vi "Timer.vi"(8 "error in (no error)":errorcluster, 11 "Message Queues in":T1) -> (0 "error out":errorcluster, 3 "Message Queue":refnum<queue>)   [LabVIEW 2014]
uses:
  support/Message Queue/All Message Queues.ctl
  support/Message Queue/Message Cluster.ctl
  Engine/Message.ctl
  support/Message Queue/Enqueue Message (Single).vi
  <vilib>/Utility/error.llb/Error Cluster From Error Code.vi
  <vilib>/ErrorRing/Error Ring.xnode
  support/Message Queue/Message Queue.lvlib
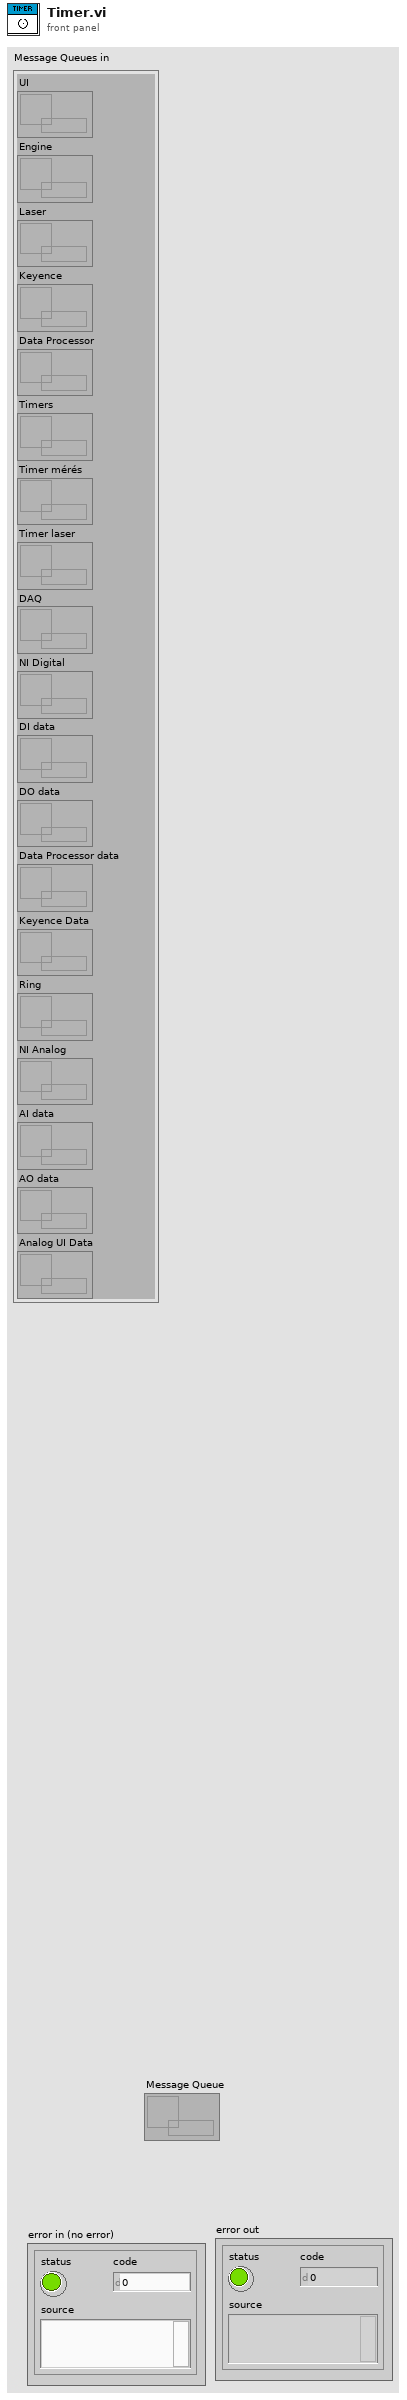
[diagram p1: front panel]
types:
  T1 = typedef "Message Queue.lvlib/All Message Queues.ctl" = cluster{"UI":refnum<queue>, "Engine":refnum<queue>, "Laser":refnum<queue>, "Keyence":refnum<queue>, "Data Processor":refnum<queue>, "Timers":refnum<queue>, "Timer mérés":refnum<queue>, "Timer laser":refnum<queue>, "DAQ":refnum<queue>, "NI Digital":refnum<queue>, "DI data":refnum<queue>, "DO data":refnum<queue>, "Data Processor data":refnum<queue>, "Keyence Data":refnum<queue>, "Ring":refnum<queue>, "NI Analog":refnum<queue>, "AI data":refnum<queue>, "AO data":refnum<queue>, "Analog UI Data":refnum<queue>}
  T2 = typedef "Message.ctl" = cluster{"Thread ID":u16, "Callback":string, "Data":variant, "Error":errorcluster}
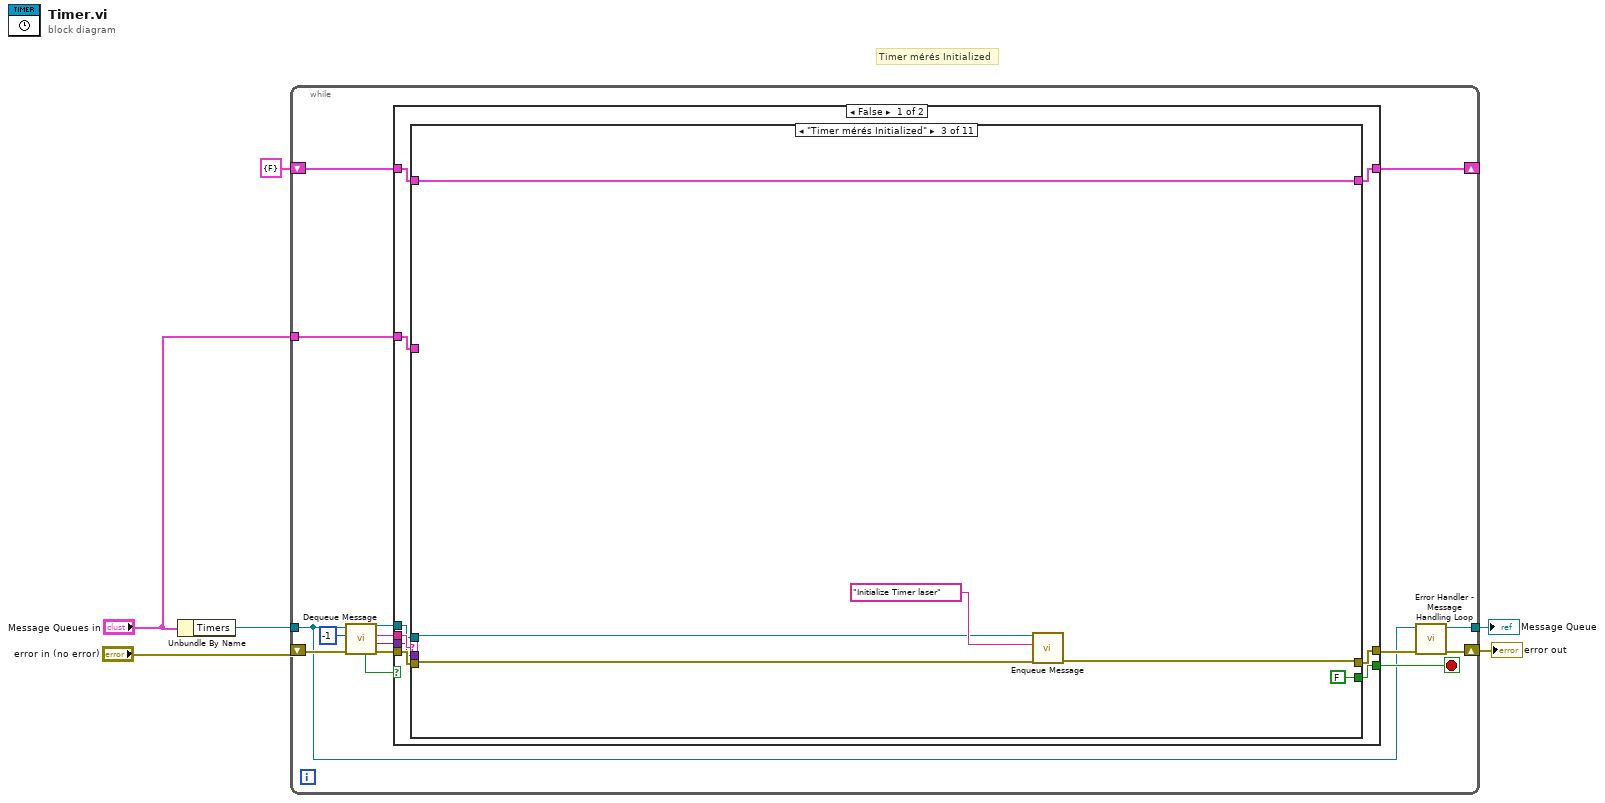
[diagram p0: block diagram]
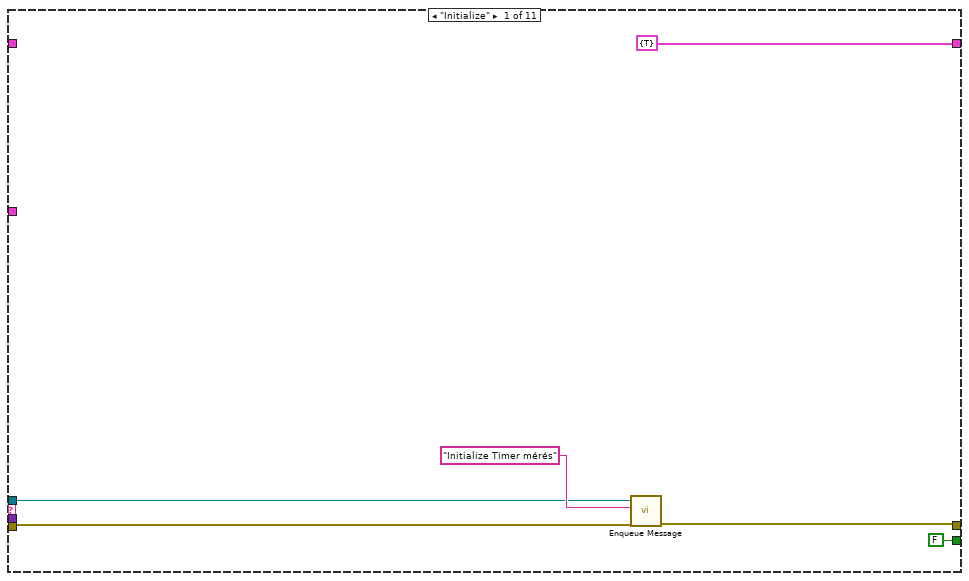
[diagram p2: hidden frame]
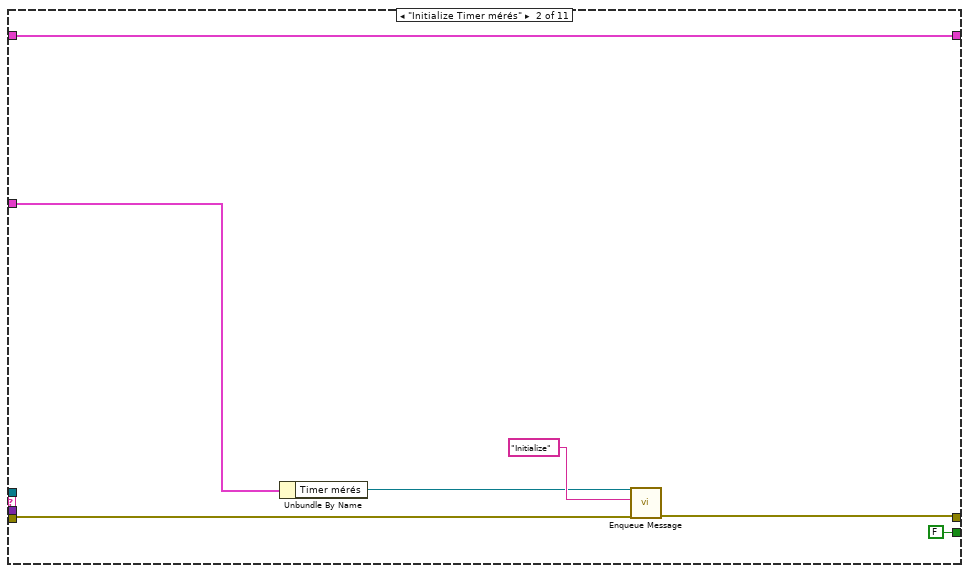
[diagram p3: hidden frame]
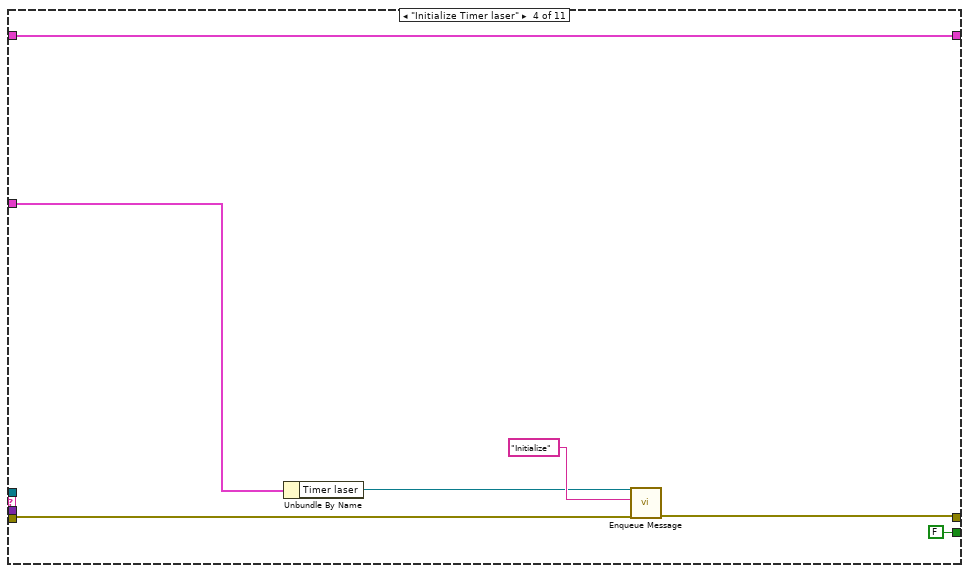
[diagram p4: hidden frame]
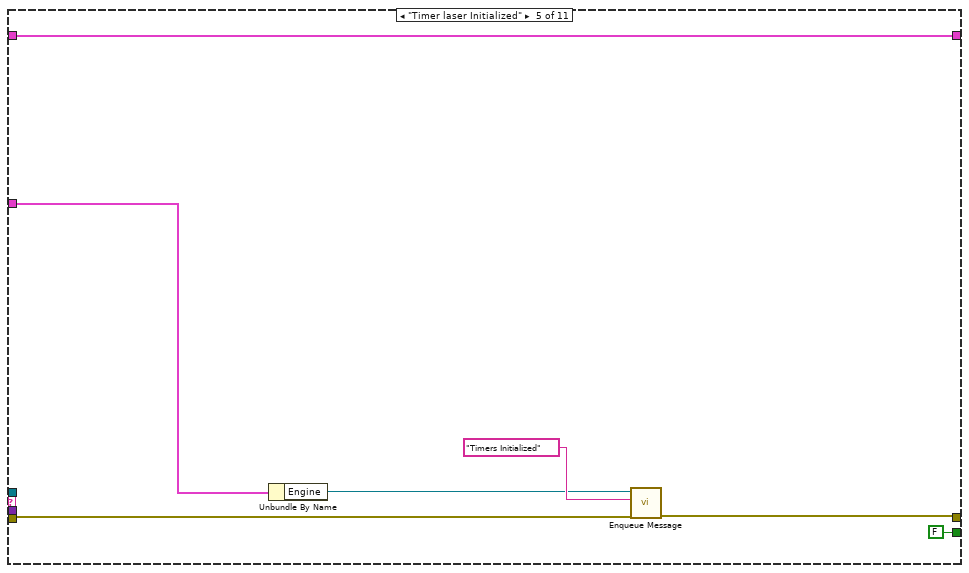
[diagram p5: hidden frame]
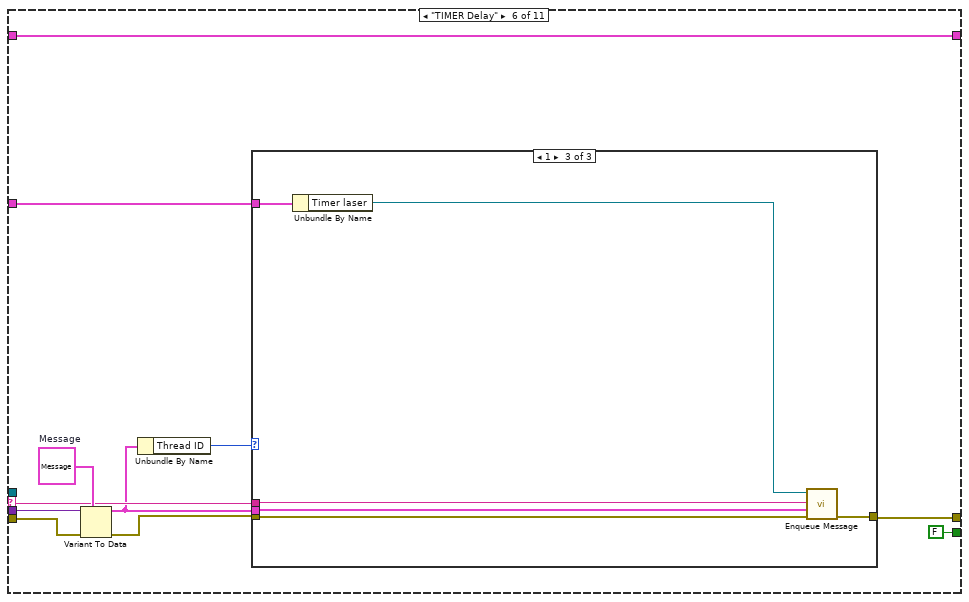
[diagram p6: hidden frame]
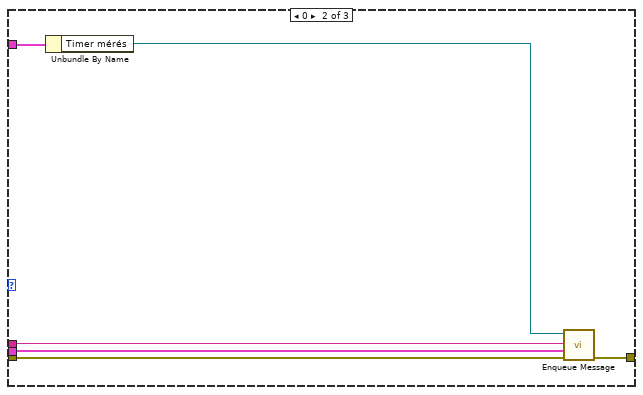
[diagram p8: hidden frame]
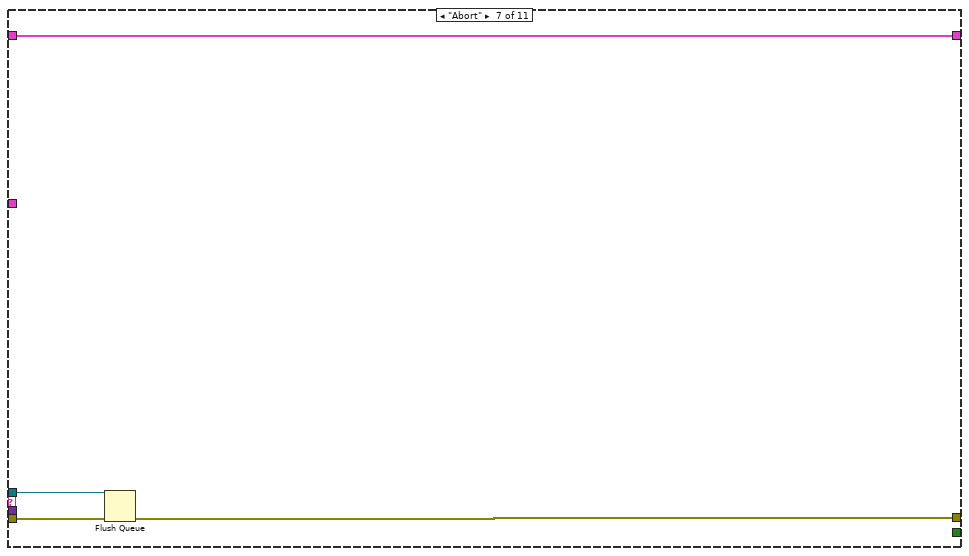
[diagram p9: hidden frame]
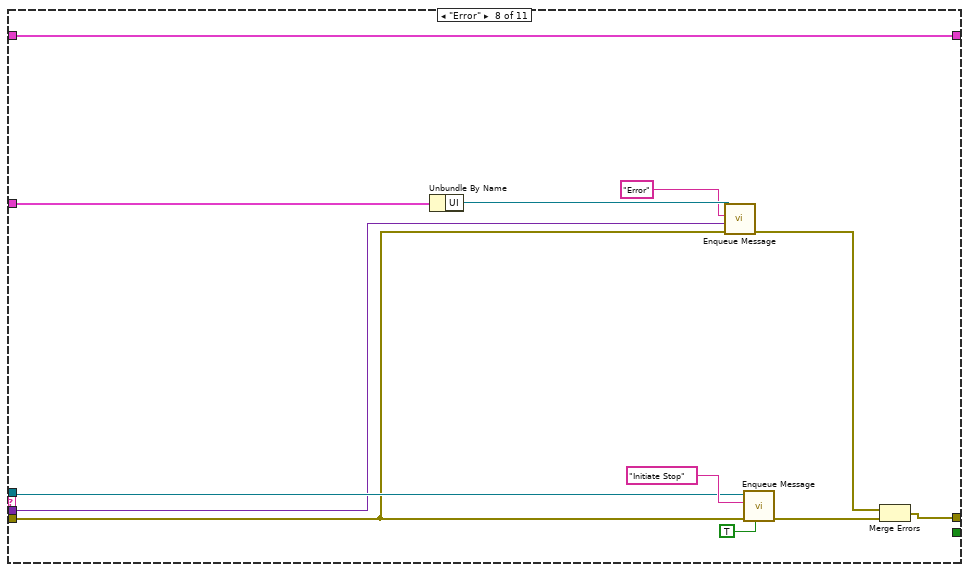
[diagram p10: hidden frame]
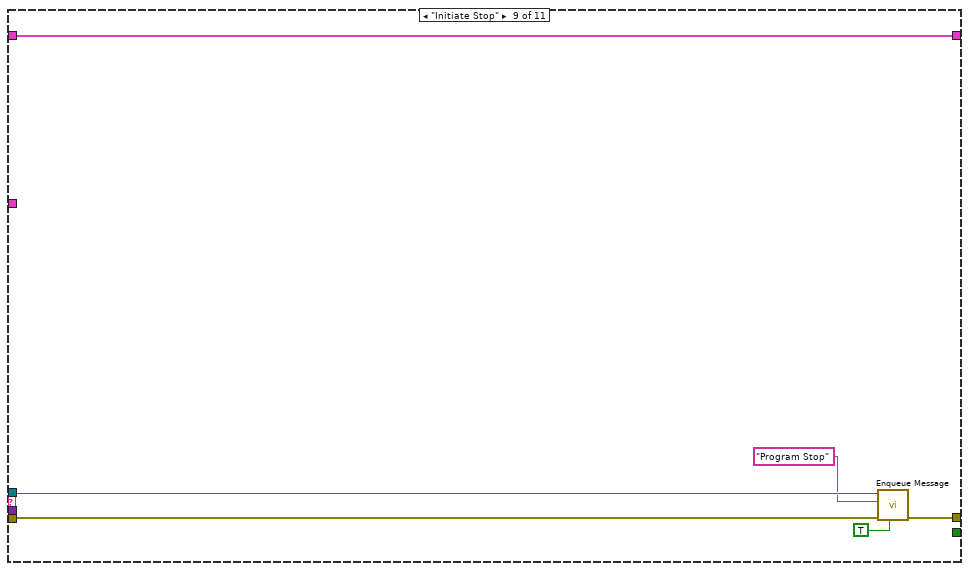
[diagram p11: hidden frame]
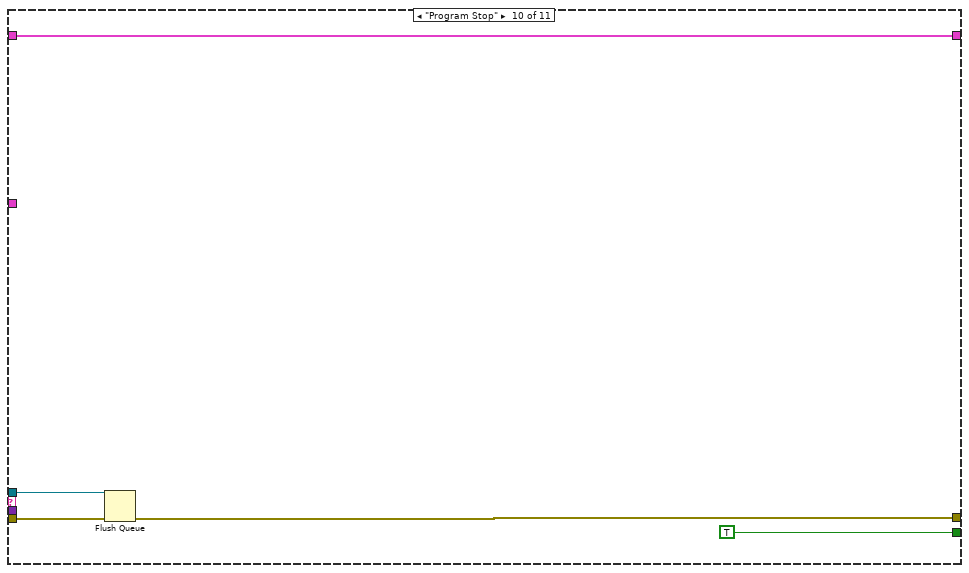
[diagram p12: hidden frame]
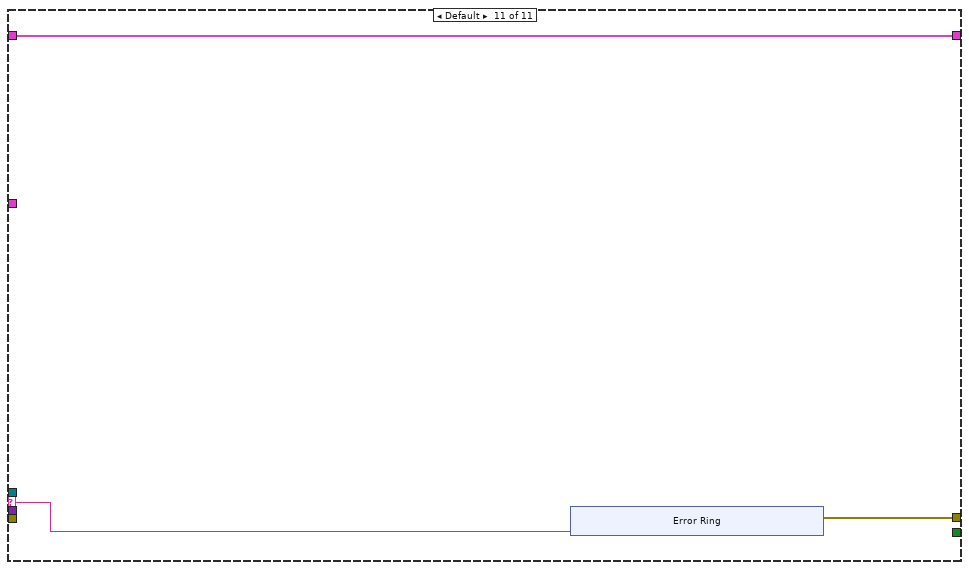
[diagram p13: hidden frame]
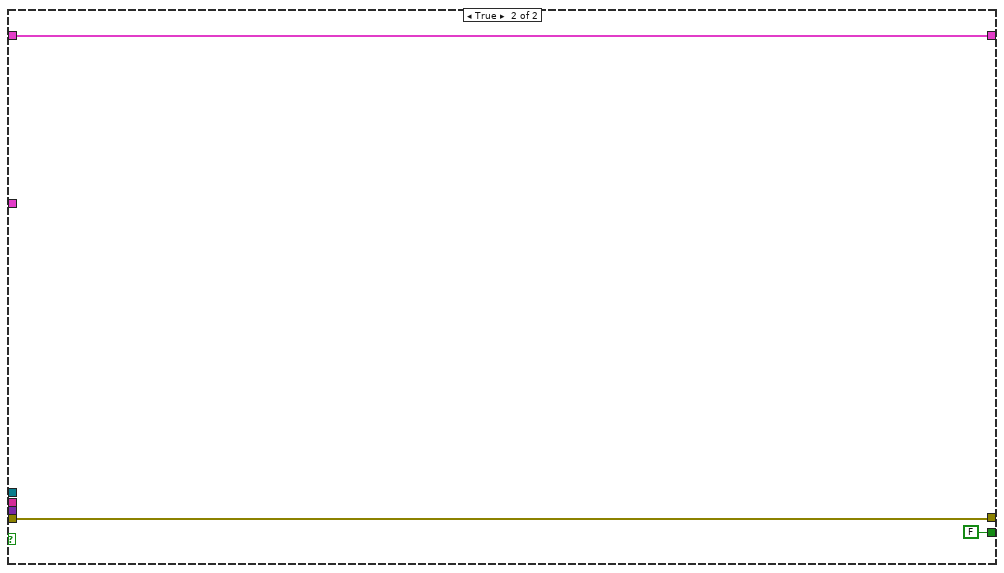
[diagram p14: hidden frame]
diagram:
  # "Timer mérés Initialized"
  n1 = Unbundle By Name("Message Queues in") -> ("Timers"=w3:refnum<queue>)
  n2 = while {
    tunnel: w3 -> [w8]
    shift-right: [w13] -> _
    shift-left: cluster{bool} {FALSE} -> [w14]
    shift-right: [w11] -> w6
    shift-left: "error in (no error)" -> [w21]
    tunnel: "Message Queues in" -> [w9]
    tunnel: [w7] -> w2
    stop <- w17 stop-if-true
    n3 = call "Dequeue Message.vi"("error in (no error)"=w21, "timeout in ms (-1)"=-1, "Message Queue"=w8) -> ("error out"=w19:errorcluster, "Message Data"=w12:variant, "Message"=w20:string, "dup Message Queue"=w18:refnum<queue>, "timed out?"=w15:bool)  [unwired: 4 in]
    n4 = case shown="False" w15 {
      tunnel: w20 -> [w30 _]
      tunnel: w19 -> [w29 w126]
      tunnel: w18 -> [w28 _]
      tunnel: [w27 FALSE] -> w17
      tunnel: [w26 w126] -> w10
      tunnel: w14 -> [w24 w127]
      tunnel: [w25 w127] -> w13
      tunnel: w12 -> [w23 _]
      tunnel: w9 -> [w22 _]
      frame False {
        n5 = case shown="\"Timer mérés Initialized\"" w30 {
          selector: w30 -> [_ _ _ _ _ w65 _ _ _ _ w115]
          tunnel: w29 -> [w33 w40 w46 w53 w60 w74 w91 w93 w107 w114 _]
          tunnel: w28 -> [w31 _ w44 _ _ _ w90 w95 w106 w113 _]
          tunnel: [w34 w41 w47 w54 w61 w67 w88 w96 w108 w110 w116] -> w26
          tunnel: [FALSE FALSE FALSE FALSE FALSE FALSE _ _ _ TRUE _] -> w27
          tunnel: [cluster{bool} {TRUE} w37 w45 w50 w59 w73 w89 w103 w109 w111 w117] -> w25
          tunnel: w24 -> [_ w37 w45 w50 w59 w73 w89 w103 w109 w111 w117]
          tunnel: w23 -> [_ _ _ _ _ w71 _ w92 _ _ _]
          tunnel: w22 -> [_ w38 _ w51 w57 w69 _ w94 _ _ _]
          frame "Initialize" {
            n6 = call-poly "Enqueue Message.vi"("error in (no error)"=w33, "Message"="Initialize Timer mérés", "Message Queue"=w31) -> ("error out"=w34:errorcluster)  [unwired: 7 in, 1 out]
          }
          frame "Initialize Timer mérés" {
            n7 = Unbundle By Name(w38) -> ("Timer mérés"=w39:refnum<queue>)
            n8 = call-poly "Enqueue Message.vi"("error in (no error)"=w40, "Message"="Initialize", "Message Queue"=w39) -> ("error out"=w41:errorcluster)  [unwired: 7 in, 1 out]
          }
          frame "Timer mérés Initialized" {
            n9 = call-poly "Enqueue Message.vi"("error in (no error)"=w46, "Message"="Initialize Timer laser", "Message Queue"=w44) -> ("error out"=w47:errorcluster)  [unwired: 7 in, 1 out]
          }
          frame "Initialize Timer laser" {
            n10 = Unbundle By Name(w51) -> ("Timer laser"=w52:refnum<queue>)
            n11 = call-poly "Enqueue Message.vi"("error in (no error)"=w53, "Message"="Initialize", "Message Queue"=w52) -> ("error out"=w54:errorcluster)  [unwired: 7 in, 1 out]
          }
          frame "Timer laser Initialized" {
            n12 = Unbundle By Name(w57) -> ("Engine"=w58:refnum<queue>)
            n13 = call-poly "Enqueue Message.vi"("error in (no error)"=w60, "Message"="Timers Initialized", "Message Queue"=w58) -> ("error out"=w61:errorcluster)  [unwired: 7 in, 1 out]
          }
          frame "TIMER Delay" {
            w70 = T2 {"Thread ID"=0, "Callback"="", "Data"=variant, "Error"={"status"=FALSE, "code"=0, "source"=""}}  # Message
            n14 = Variant To Data(error in=w74, type=w70, Variant=w71) -> (data=w64:T2, error out=w66:errorcluster)
            n15 = Unbundle By Name(w64) -> ("Thread ID"=w68:u16)
            n16 = case shown="1" w68 {
              tunnel: w69 -> [_ w81 w87]
              tunnel: [w75 w80 w86] -> w67
              tunnel: w66 -> [w75 w76 w82]
              tunnel: w65 -> [_ w78 w84]
              tunnel: w64 -> [_ w77 w83]
              frame Default {
              }
              frame 0 {
                n17 = Unbundle By Name(w81) -> ("Timer mérés"=w79:refnum<queue>)
                n18 = call-poly "Enqueue Message.vi"("error in (no error)"=w76, "Message Data"=w77, "Message"=w78, "Message Queue"=w79) -> ("error out"=w80:errorcluster)  [unwired: 6 in, 1 out]
              }
              frame 1 {
                n19 = Unbundle By Name(w87) -> ("Timer laser"=w85:refnum<queue>)
                n20 = call-poly "Enqueue Message.vi"("error in (no error)"=w82, "Message Data"=w83, "Message"=w84, "Message Queue"=w85) -> ("error out"=w86:errorcluster)  [unwired: 6 in, 1 out]
              }
            }
          }
          frame "Abort" {
            n21 = Flush Queue(queue=w90, error in (no error)=w91) -> (error out=w88:errorcluster)  [unwired: 2 out]
          }
          frame "Error" {
            n22 = Unbundle By Name(w94) -> ("UI"=w100:refnum<queue>)
            n23 = call-poly "Enqueue Message.vi"("error in (no error)"=w93, "Message Data"=w92, "Message"="Error", "Message Queue"=w100) -> ("error out"=w102:errorcluster)  [unwired: 6 in, 1 out]
            n24 = call-poly "Enqueue Message.vi"("Priority Message? (F)"=TRUE, "error in (no error)"=w93, "Message"="Initiate Stop", "Message Queue"=w95) -> ("error out"=w101:errorcluster)  [unwired: 6 in, 1 out]
            n25 = Merge Errors(w102, w101) -> (w96:errorcluster)
          }
          frame "Initiate Stop" {
            n26 = call-poly "Enqueue Message.vi"("Priority Message? (F)"=TRUE, "error in (no error)"=w107, "Message"="Program Stop", "Message Queue"=w106) -> ("error out"=w108:errorcluster)  [unwired: 6 in, 1 out]
          }
          frame "Program Stop" {
            n27 = Flush Queue(queue=w113, error in (no error)=w114) -> (error out=w110:errorcluster)  [unwired: 2 out]
          }
          frame Default {
            n28 = xnode "Error Ring"("parameter 0"=w115) -> ("error out"=w116:errorcluster)
          }
        }
      }
      frame True {
      }
    }
    n29 = call "Error Handler - Message Handling Loop.vi"("error in (no error)"=w10, "Message Queue"=w8) -> ("dup error in"=w11:errorcluster, "dup Message Queue"=w7:refnum<queue>)  [unwired: 8 in]
  }
  "error out" <- w6
  "Message Queue" <- w2
